vi "Synthetic_Jet_LDA.vi"() -> (5 "Plug in titles":string[](array[string]), 7 "Plug in values":string[](array[string]))   [LabVIEW 2011]
uses:
  Controls/SJ_Data_Cluster.ctl
  Controls/SJ_Results_Cluster.ctl
  Controls/SJ_Channels.ctl
  Controls/Post_Process.ctl
  Globals/Meas_global.vi
  <vilib>/Analysis/1siggen.llb/Ramp Pattern by Delta.vi
  <vilib>/Analysis/NI_AALBase.lvlib
  <vilib>/gmath/NI_Gmath.lvlib
panel:
  in  "Number of Bins":i32=30
  out "SJ Results Array":T1[](array[typedef])=[{"Phase"=[], "Phase Averaged"=[], "RMS Value"=8.35157278710812, "Channel Name"="LDA (U)", "Max Value"=0.0, "Phase Angle"=1.0, "Jet Frequency"=1039.7638647645044, "Samples/Bin"=0, "Phase Plot"={"Phase Angle"=[], []}}, {"Phase"=[], "Phase Averaged"=[], "RMS Value"=2.779220166180465, "Channel Name"="LDA (V)", "Max Value"=0.0, "Phase Angle"=1.0, "Jet Frequency"=1039.7638647645044, "Samples/Bin"=0, "Phase Plot"={"Phase Angle"=[], []}}, {"Phase"=[], "Phase Averaged"=[nan], "RMS Value"=2.785281670112028, "Channel Name"="RV (Sync)", "Max Value"=0.0, "Phase Angle"=nan, "Jet Frequency"=1039.7638647645044, "Samples/Bin"=0, "Phase Plot"={"Phase Angle"=[], [nan]}}, {"Phase"=[], "Phase Averaged"=[nan], "RMS Value"=1.4716860650069226, "Channel Name"="RV (Vin)", "Max Value"=0.0, "Phase Angle"=nan, "Jet Frequency"=1039.7638647645044, "Samples/Bin"=0, "Phase Plot"={"Phase Angle"=[], [nan]}}, {"Phase"=[], "Phase Averaged"=[nan], "RMS Value"=0.24568070029652622, "Channel Name"="RV (HW)", "Max Value"=0.0, "Phase Angle"=nan, "Jet Frequency"=1039.7638647645044, "Samples/Bin"=0, "Phase Plot"={"Phase Angle"=[], [nan]}}]
  out "Dwell Time":u32=200
  out "Analogue Sampling Rate":dbl=40000.0
  out "No of Analogue Samples":i32=40000
  out "Analogue Aquisition Time":dbl=999.975
  out "Analogue Samples":i32=39999
  out "dt":dbl=inf
  out "No of bins":i32
  out "Analogue Fs":dbl=40000.0
  out "Current Block No":i32=25
  out "Next Frequency":dbl=1060.0
  out "Zero Values":dbl[](array[numeric])=[0.0030001498508715582, 0.0061511235517187676, 2.208881239967972, 0.0008108304920773175, 1.5203627177178738]
  out "SJ Data":T2={"Do"=0.005, "Dc"=0.038, "Ho"=0.01, "Hc"=0.008, "K"=1.14, "beta"=0.424, "Vc"=2.0, "Vo"=2.375}
  out "Current Frequency":dbl=1039.7638647645044 format="%0.4f"
  out "Frequency Array":dbl[](array[numeric])=[600.0, 620.0, 640.0, 660.0, 680.0, 700.0, 720.0, 740.0, 760.0, 780.0, 800.0, 820.0, 840.0, 860.0, 880.0, 900.0, 920.0, 940.0, 960.0, 980.0, 1000.0, 1020.0, 1040.0, 1060.0, 1080.0, 1100.0, 1120.0, 1140.0, 1160.0, 1180.0, 1200.0]
  # "You Must have selected the \"Save Data\" option on the \nMeasurement Program for this vi to work correctly"
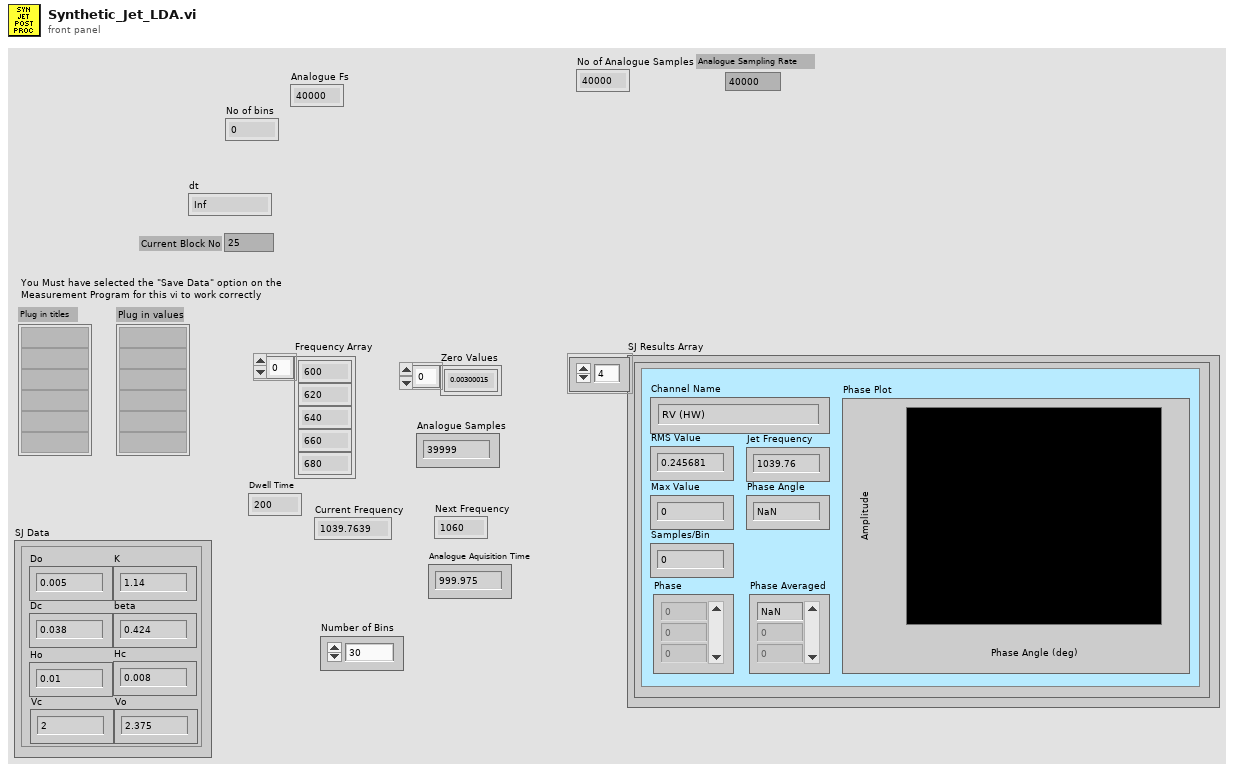
[diagram p1: front panel]
types:
  T1 = typedef "SJ_Results_Cluster.ctl" = cluster{"Phase":dbl[], "Phase Averaged":dbl[], "RMS Value":dbl, "Channel Name":string, "Max Value":dbl, "Phase Angle":dbl, "Jet Frequency":dbl, "Samples/Bin":i32, "Phase Plot":cluster{"Phase Angle":dbl[], dbl[]}}
  T2 = typedef "SJ_Data_Cluster.ctl" = cluster{"Do":dbl, "Dc":dbl, "Ho":dbl, "Hc":dbl, "K":dbl, "beta":dbl, "Vc":dbl, "Vo":dbl}
  T3 = typedef "SJ_Channels.ctl" = string[]
  T4 = typedef "Analysis_info_cluster.ctl" = cluster{"Colour":u32, "Inst type":T5, "Inst name":string, "Symbol":string, "Code name":string, "Extra Info":string, "Inst Array":T6, "Index":i32, "Voltage Index":i32, "Extra Titles":string[], "Extra Values":string[], "Eng Values":dbl[], "Time (ms)":dbl[], "TT / Voltage":dbl[], "U":dbl, "u^2":dbl, "u^3":dbl, "u^4":dbl, "Skew_u":dbl, "Kurt_u":dbl, "Mean % Err":dbl, "% u'/U":dbl}
  T5 = typedef "Inst_type.ctl" = enum16{"Propeller anemometer", "Raw voltage", "Pressure Transducer", "Pitot-static tube", "Preston tube", "Hot wire", "Cross wire 1", "Cross wire 2", "Generic Linear", "Generic Polynomial", "Generic BackPoly", "Fast FID", "Thermocouple", "Cold wire", "Pulsed Wire", "LDA Vel", "LDA Tran time", "LDA Arr time"}
  T6 = typedef "Instrument_Array.ctl" = enum16{"PWA", "LDA", "Analogue"}
  T7 = typedef "Post_Process.ctl" = enum16{"Take New Data", "Post Process Raw Data File"}
  T8 = cluster{"Name":string, "X":dbl, "Y":dbl, "Z":dbl}[]
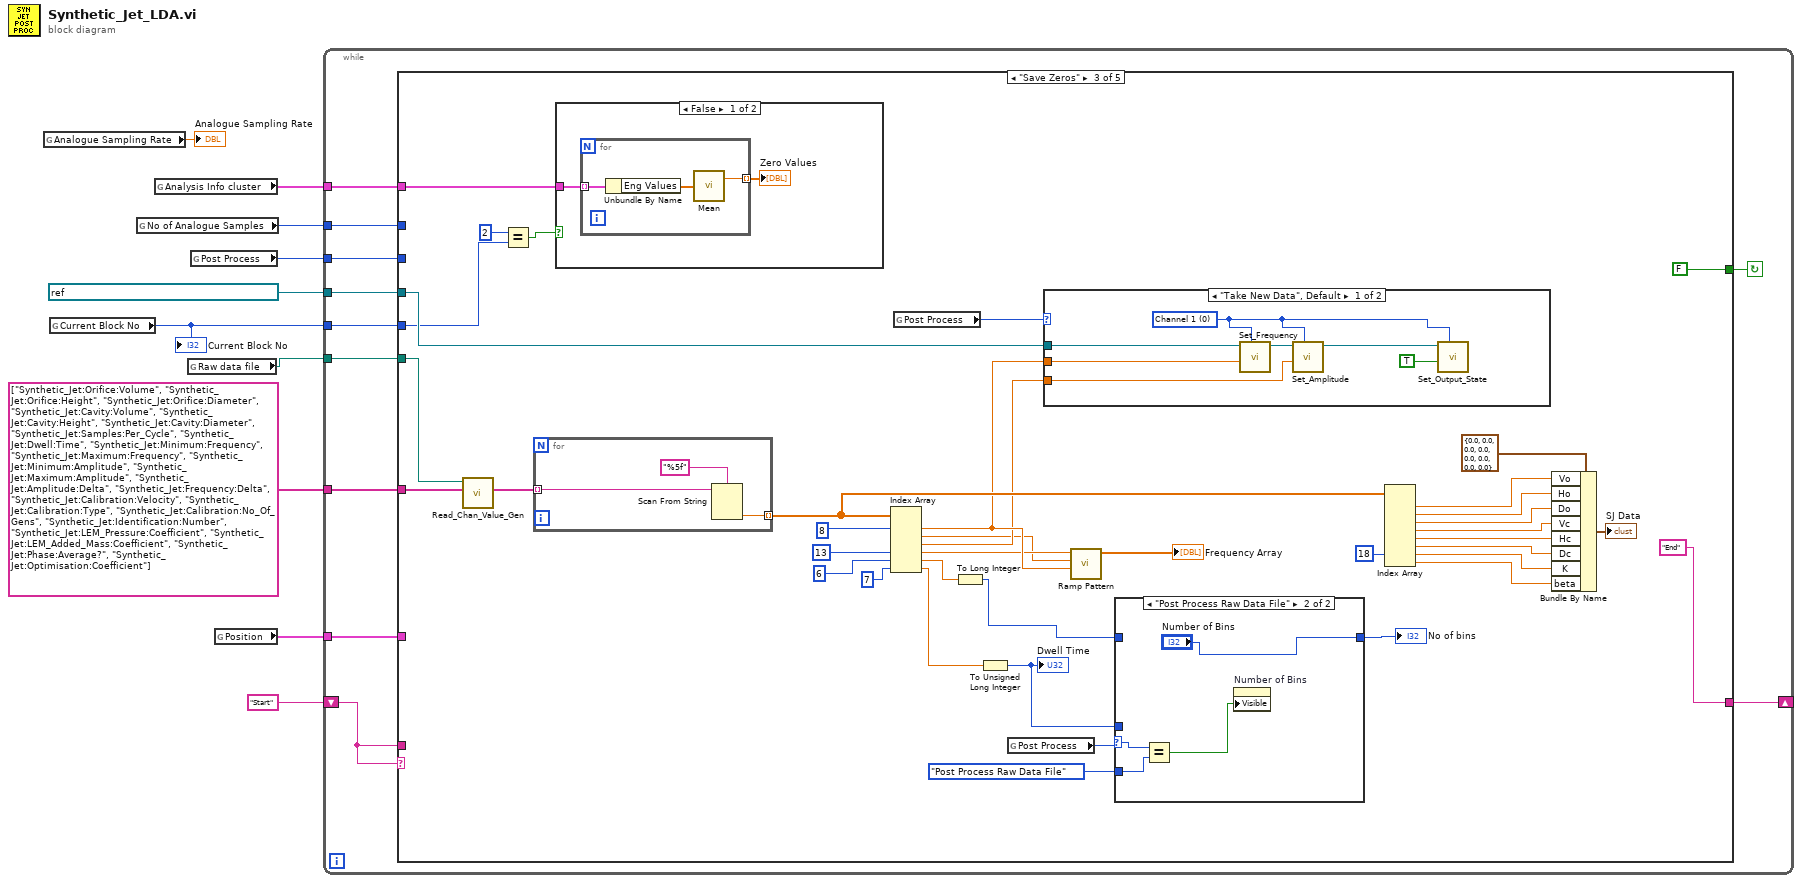
[diagram p0: block diagram]
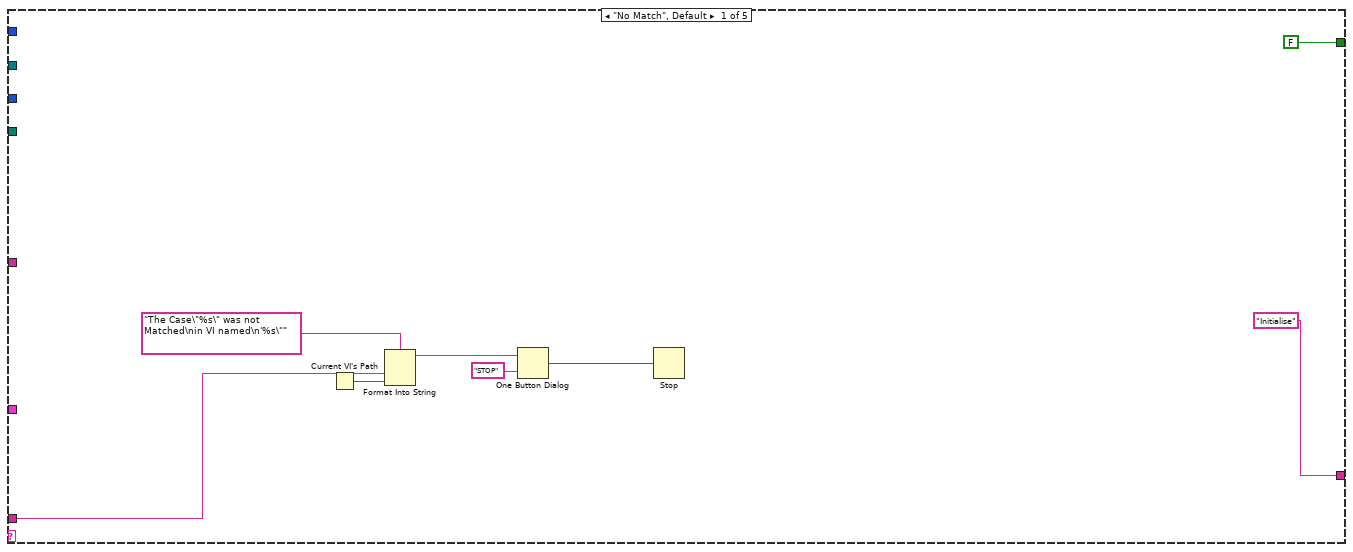
[diagram p2: hidden frame]
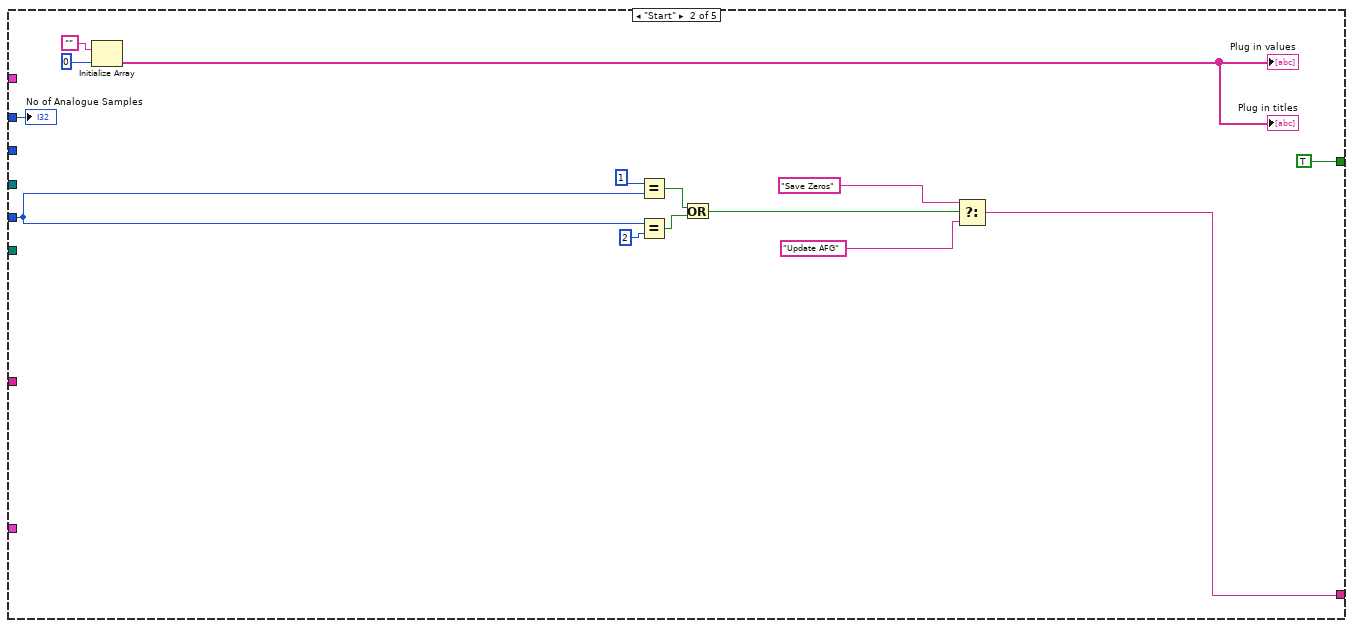
[diagram p3: hidden frame]
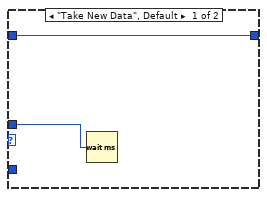
[diagram p4: hidden frame]
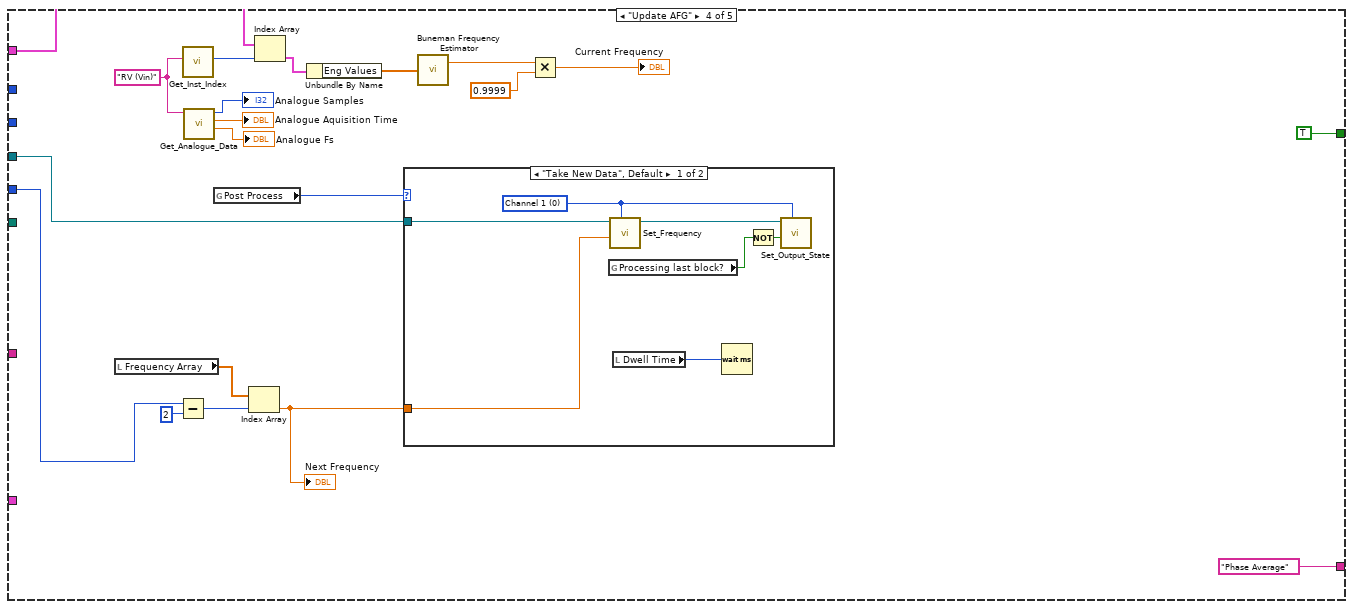
[diagram p7: hidden frame]
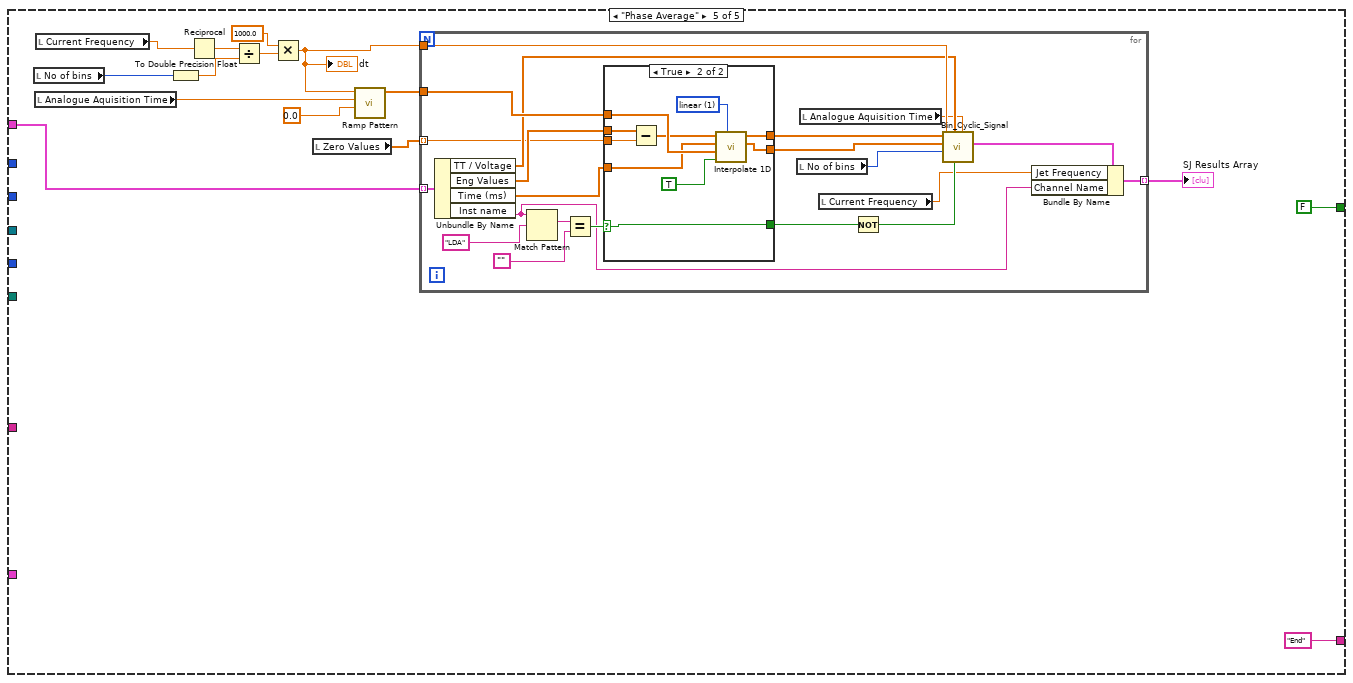
[diagram p9: hidden frame]
diagram:
  n1 = global read "Meas_global.vi" "Analogue Sampling Rate"() -> (→"Analogue Sampling Rate":dbl)
  n2 = global read "Meas_global.vi" "Current Block No"() -> (w8:i32)
  "Current Block No" <- w8
  n3 = global read "Meas_global.vi" "No of Analogue Samples"() -> (w6:i32)
  n4 = global read "Meas_global.vi" "Analysis Info cluster"() -> (w7:T4[])
  n5 = global read "Meas_global.vi" "Raw data file"() -> (w9:path)
  n6 = global read "Meas_global.vi" "Post Process"() -> (w4:T7)
  n7 = global read "Meas_global.vi" "Position"() -> (w5:T8)
  n8 = while {
    shift-left: "Start" -> [w21]
    shift-right: [w15] -> _
    tunnel: w9 -> [w20]
    tunnel: w8 -> [w16]
    tunnel: w7 -> [w19]
    tunnel: w6 -> [w18]
    tunnel: w5 -> [w17]
    tunnel: w4 -> [w13]
    tunnel: T3 ["Synthetic_Jet:Orifice:Volume", "Synthetic_Jet:Orifice:Height", "Synthetic_Jet:Orifice:Diameter", "Synthetic_Jet:Cavity:Volume", "Synthetic_Jet:Cavity:Height", "Synthetic_Jet:Cavity:Diameter", "Synthetic_Jet:Samples:Per_Cycle", "Synthetic_Jet:Dwell:Time", "Synthetic_Jet:Minimum:Frequency", "Synthetic_Jet:Maximum:Frequency", "Synthetic_Jet:Minimum:Amplitude", "Synthetic_Jet:Maximum:Amplitude", "Synthetic_Jet:Amplitude:Delta", "Synthetic_Jet:Frequency:Delta", "Synthetic_Jet:Calibration:Velocity", "Synthetic_Jet:Calibration:Type", "Synthetic_Jet:Calibration:No_Of_Gens", "Synthetic_Jet:Identification:Number", "Synthetic_Jet:LEM_Pressure:Coefficient", "Synthetic_Jet:LEM_Added_Mass:Coefficient", "Synthetic_Jet:Phase:Average?", "Synthetic_Jet:Optimisation:Coefficient"] ("Synthetic Jet Specific Channels") -> [w12]
    tunnel: refnum<visa-resource-name> "USB0::0x0699::0x0347::C036837::INSTR" ("VISA resource name") -> [w11]
    stop <- w14 continue-if-true
    n9 = case shown="\"Save Zeros\"" w21 {
      tunnel: w21 -> [w25 _ _ _ _]
      tunnel: w20 -> [_ _ w79 _ _]
      tunnel: w16 -> [_ w35 w56 w119 _]
      tunnel: w19 -> [_ _ w58 w113 w132]
      tunnel: w18 -> [_ w30 _ _ _]
      tunnel: w17 -> [_ _ _ _ _]
      tunnel: ["Initialise" w40 "End" ("t") "Phase Average" ("t") "End" ("t")] -> w15
      tunnel: [FALSE TRUE FALSE TRUE FALSE] -> w14
      tunnel: w13 -> [_ _ _ _ _]
      tunnel: w12 -> [_ _ w78 _ _]
      tunnel: w11 -> [_ _ w64 w116 _]
      frame "No Match", Default {
        n10 = Current VI's Path() -> (path=w24:path)
        n11 = Format Into String(format string="The Case\"%s\" was not Matched\nin VI named\n'%s\"" ("Format String"), w25, w24) -> (resulting string=w28:string)  [unwired: 2 in, 1 out]
        n12 = One Button Dialog(message=w28, button name ("OK")="STOP") -> (true=w26:bool)
        n13 = Stop(stop? (T)=w26) -> ()
      }
      frame "Start" {
        n14 = Initialize Array("", 0) -> (→"Plug in values" →"Plug in titles":string[])
        n15 = Equal?(x=1, y=w35) -> (x = y?=w33:bool)
        n16 = Equal?(x=w35, y=2 ("x")) -> (x = y?=w34:bool)
        n17 = Or(x=w33, y=w34) -> (x .or. y?=w32:bool)
        n18 = Select(t="Save Zeros", s=w32, f="Update AFG") -> (s? t:f=w40:string)
        "No of Analogue Samples" <- w30
      }
      frame "Save Zeros" {
        n19 = call "Read_Chan_Value_Gen.vi"("Desired Ch Names"=w78, "Raw data file"=w79) -> ("Values"=w68:string[])  [unwired: 9 in]
        n20 = Equal?(x=2, y=w56) -> (x = y?=w54:bool)
        n21 = for {
          tunnel: w68 -> [w103] mode=indexing
          tunnel: [w101] -> w63 mode=indexing
          n22 = Scan From String(format string="%5f", input string=w103) -> (output 1=w101:dbl)  [unwired: 3 in, 3 out]
        }
        n23 = case shown="False" w54 {
          tunnel: w58 -> [w90 _]
          frame False {
            n24 = for {
              tunnel: w90 -> [w93] mode=indexing
              tunnel: [w91] -> w89 mode=indexing
              n25 = Unbundle By Name(w93) -> ("Eng Values"=w92:dbl[])
              n26 = call <vilib>:"Mean.vi"("X"=w92) -> ("mean"=w91:dbl)  [unwired: 1 out]
            }
            "Zero Values" <- w89
          }
          frame True {
          }
        }
        n27 = Index Array(array=w63, index #1=8 ("index"), index #4=13 ("index"), index #5=6 ("index"), index #6=7 ("index")) -> (element #1=w62:dbl, element #2=w53:dbl, element #3=w61:dbl, element #4=w60:dbl, element #5=w51:dbl, element #6=w49:dbl)  [unwired: 2 in]
        n28 = global read "Meas_global.vi" "Post Process"() -> (w65:T7)
        n29 = To Long Integer(number=w51) -> (32bit integer=w46:i32)
        n30 = To Unsigned Long Integer(number=w49) -> (unsigned 32bit integer=w47:u32)
        "Dwell Time" <- w47
        n31 = global read "Meas_global.vi" "Post Process"() -> (w48:T7)
        n32 = case shown="\"Take New Data\", Default" w65 {
          tunnel: w61 -> [w100 _]
          tunnel: w62 -> [w95 _]
          tunnel: w64 -> [w94 _]
          frame "Take New Data", Default {
            w97 = u16 0 items=["Channel 1", "Channel 2"] ("Menu Ring")
            n33 = call "Set_Frequency.vi"("Menu Ring"=w97, "Frequency"=w95, "VISA resource name"=w94) -> ("VISA resource name out"=w98:refnum<visa-resource-name>)  [unwired: 8 in]
            n34 = call "Set_Amplitude.vi"("Menu Ring 2"=w97, "Amplitude"=w100, "VISA resource name"=w98) -> ("VISA resource name out"=w99:refnum<visa-resource-name>)  [unwired: 8 in]
            n35 = call "Set_Output_State.vi"("Menu Ring"=w97, "Output State"=TRUE, "VISA resource name"=w99) -> ()  [unwired: 9 in]
          }
          frame "Post Process Raw Data File" {
          }
        }
        n36 = call-poly <vilib>:"Ramp Pattern.vi"("start"=w62, "end"=w53, "delta"=w60) -> ("Ramp Pattern"=→"Frequency Array":dbl[])  [unwired: 6 in, 2 out]
        n37 = case shown="\"Post Process Raw Data File\"" w48 {
          selector: w48 -> [_ w88]
          tunnel: w47 -> [w84 _]
          tunnel: w46 -> [w83 _]
          tunnel: Post_Process."Post Process Raw Data File" ("Post Process") -> [_ w87]
          tunnel: [w83 "Number of Bins"] -> w44
          frame "Take New Data", Default {
            n38 = Wait (ms)(milliseconds to wait=w84) -> ()  [unwired: 1 out]
          }
          frame "Post Process Raw Data File" {
            n39 = Equal?(x=w88, y=w87) -> (x = y?=w85:bool)
            n40 = property on="Number of Bins" class="DigNum (strict)"("Visible"=w85) -> ()  [unwired: 2 in, 2 out]
          }
        }
        "No of bins" <- w44
        n41 = Index Array(array=w63, index #7=18 ("index")) -> (element #1=w77:dbl, element #2=w76:dbl, element #3=w75:dbl, element #4=w74:dbl, element #5=w73:dbl, element #6=w72:dbl, element #7=w70:dbl, element #8=w69:dbl)  [unwired: 7 in]
        n42 = Bundle By Name(cluster=T2 {"Do"=0.0, "Dc"=0.0, "Ho"=0.0, "Hc"=0.0, "K"=0.0, "beta"=0.0, "Vc"=0.0, "Vo"=0.0} ("SJ_Data_Cluster"), "Vo"=w77, "Ho"=w76, "Do"=w75, "Vc"=w74, "Hc"=w73, "Dc"=w72, "K"=w70, "beta"=w69) -> (→"SJ Data":T2)
      }
      frame "Update AFG" {
        w114 = "RV (Vin)" ("Inst name search")
        n43 = local read "Frequency Array"() -> (w122:dbl[])
        n44 = Subtract(x=w119, y=2) -> (x-y=w121:i32)
        n45 = call "Get_Inst_Index.vi"("Inst name search"=w114) -> ("Index of Instance"=w112:i32)  [unwired: 8 in, 2 out]
        n46 = call "Get_Analogue_Data.vi"("Inst (Inst 2 if blank)"=w114) -> ("Analogue Fs"=→"Analogue Fs":dbl, "Analogue Aquasition Time"=→"Analogue Aquisition Time":dbl, "Analogue Samples"=→"Analogue Samples":i32)  [unwired: 8 in]
        n47 = global read "Meas_global.vi" "Post Process"() -> (w117:T7)
        n48 = Index Array(array=w122, index=w121) -> (element=w118:dbl)
        "Next Frequency" <- w118
        n49 = Index Array(array=w113, index=w112) -> (element=w111:T4)
        n50 = Unbundle By Name(w111) -> ("Eng Values"=w105:dbl[])
        n51 = case shown="\"Take New Data\", Default" w117 {
          tunnel: w118 -> [w129 _]
          tunnel: w116 -> [w127 _]
          frame "Take New Data", Default {
            w130 = u16 0 items=["Channel 1", "Channel 2"] ("Menu Ring")
            n52 = global read "Meas_global.vi" "Processing last block?"() -> (w125:bool)
            n53 = call "Set_Frequency.vi"("Menu Ring"=w130, "Frequency"=w129, "VISA resource name"=w127) -> ("VISA resource name out"=w128:refnum<visa-resource-name>)  [unwired: 8 in]
            n54 = local read "Dwell Time"() -> (w124:u32)
            n55 = Wait (ms)(milliseconds to wait=w124) -> ()  [unwired: 1 out]
            n56 = Not(x=w125) -> (.not. x?=w126:bool)
            n57 = call "Set_Output_State.vi"("Menu Ring"=w130, "Output State"=w126, "VISA resource name"=w128) -> ()  [unwired: 9 in]
          }
          frame "Post Process Raw Data File" {
          }
        }
        n58 = call <vilib>:"Buneman Frequency Estimator.vi"("X"=w105) -> ("beta"=w104:dbl)  [unwired: 1 out]
        n59 = Multiply(x=w104, y=0.9999) -> (x*y=→"Current Frequency":dbl)
      }
      frame "Phase Average" {
        n60 = local read "No of bins"() -> (w140:i32)
        n61 = local read "Analogue Aquisition Time"() -> (w139:dbl)
        n62 = local read "Current Frequency"() -> (w136:dbl)
        n63 = To Double Precision Float(number=w140) -> (double precision float=w143:dbl)
        n64 = Reciprocal(x=w136) -> (1/x=w142:dbl)
        n65 = Divide(x=w142, y=w143) -> (x/y=w138:dbl)
        n66 = Multiply(x=1000.0, y=w138) -> (x*y=w134:dbl)
        "dt" <- w134
        n67 = local read "Zero Values"() -> (w133:dbl[])
        n68 = call-poly <vilib>:"Ramp Pattern.vi"("start"=0.0, "end"=w139, "delta"=w134) -> ("Ramp Pattern"=w135:dbl[])  [unwired: 6 in, 2 out]
        n69 = for {
          tunnel: w135 -> [w155]
          tunnel: w134 -> [w154]
          tunnel: w133 -> [w151] mode=indexing
          tunnel: w132 -> [w150] mode=indexing
          tunnel: [w146] -> w131 mode=indexing
          n70 = Unbundle By Name(w150) -> ("TT / Voltage"=w153:dbl[], "Eng Values"=w161:dbl[], "Time (ms)"=w162:dbl[], "Inst name"=w148:string)
          n71 = Match Pattern(string=w148, regular expression="LDA") -> (match substring=w165:string)  [unwired: 1 in, 3 out]
          n72 = Equal?(x=w165, y="") -> (x = y?=w163:bool)
          n73 = case shown="True" w163 {
            selector: w163 -> [w167 w173]
            tunnel: w155 -> [_ w178]
            tunnel: w162 -> [w168 w177]
            tunnel: w161 -> [w169 w172]
            tunnel: [w169 w175] -> w160
            tunnel: [w168 w174] -> w159
            tunnel: [w167 w173] -> w158
            tunnel: w151 -> [_ w170]
            frame False {
            }
            frame True {
              w179 = 1 items=["nearest", "linear", "spline", "cubic Hermite", "Lagrange"] ("method")
              n74 = Subtract(x=w172, y=w170) -> (x-y=w171:dbl[])
              n75 = call <vilib>:"Interpolate 1D.vi"("method"=w179, "X is monotonic"=TRUE, "xi"=w178, "X"=w177, "Y"=w171) -> ("xi used"=w174:dbl[], "yi"=w175:dbl[])  [unwired: 4 in, 1 out]
            }
          }
          n76 = local read "No of bins"() -> (w156:i32)
          n77 = local read "Analogue Aquisition Time"() -> (w152:dbl)
          n78 = local read "Current Frequency"() -> (w147:dbl)
          n79 = Not(x=w158) -> (.not. x?=w157:bool)
          n80 = call "Bin_Cyclic_Signal.vi"("Max Time"=w152, "LDA Data? (False)"=w157, "Transit Time"=w153, "dt"=w154, "No of bins"=w156, "Time"=w159, "Eng Values"=w160) -> ("SJ Results"=w149:T1)  [unwired: 4 in]
          n81 = Bundle By Name(cluster=w149, "Jet Frequency"=w147, "Channel Name"=w148) -> (w146:T1)
        }
        "SJ Results Array" <- w131
      }
    }
  }
